vi "SendOracleRequest.vi"(8 "error in (no error)":errorcluster, 9 "Timeout":i32=5000, 10 "Report End Date":timestamp, 11 "Report Start Date":timestamp) -> (0 "error out":errorcluster, 3 "String":string)   [LabVIEW 2018, in "Controller.lvlib"]
uses:
  Controller.lvlib
  SRDataManagement_1.0/MainFrame/MainFrameLib.lvlib
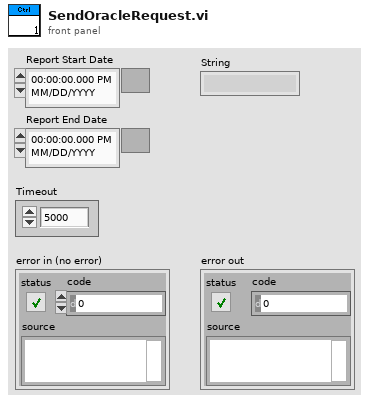
[diagram p1: front panel]
types:
  T1 = enum16{"Read", "Write", "ReadWrite", "BufferedRead", "BufferedReadWrite"}
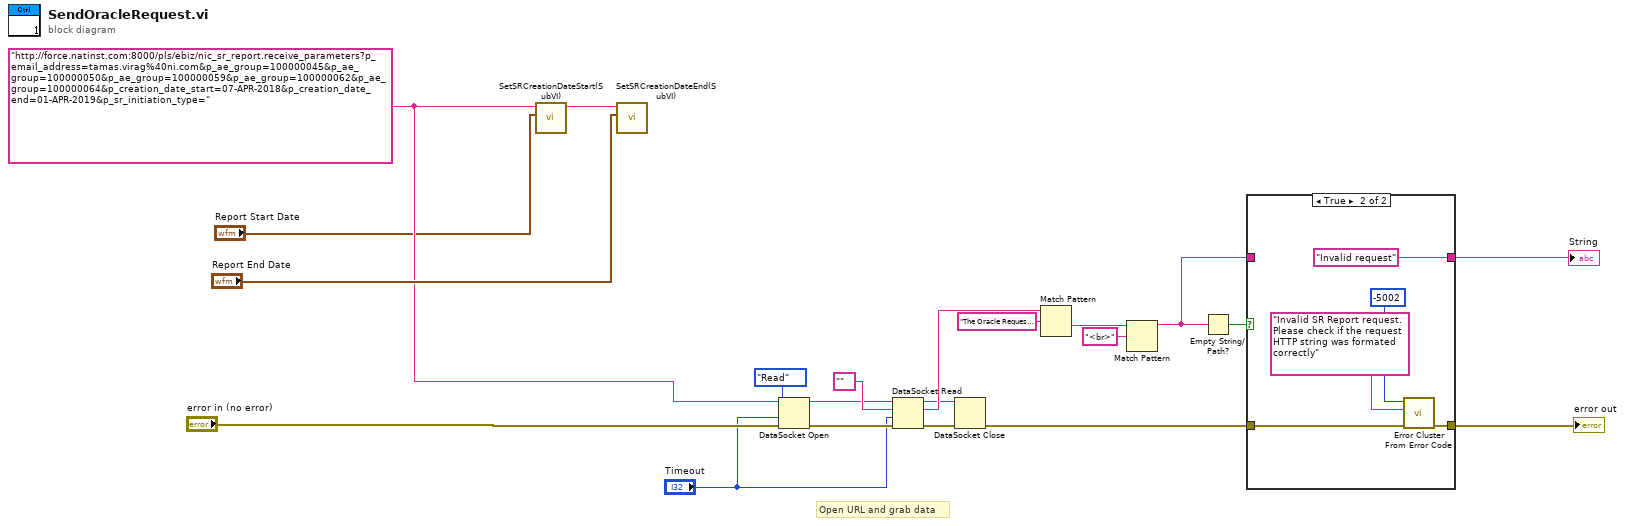
[diagram p0: block diagram]
diagram:
  w2 = "http://force.natinst.com:8000/pls/ebiz/nic_sr_report.receive_parameters?p_email_address=tamas.virag%40ni.com&p_ae_group=100000045&p_ae_group=100000050&p_ae_group=100000059&p_ae_group=100000062&p_ae_group=100000064&p_creation_date_start=07-APR-2018&p_creation_date_end=01-APR-2019&p_sr_initiation_type=" ("HTTP string")
  # "Open URL and grab data"
  n1 = call "SetSRCreationDateStart(SubVI).vi"("Date"="Report Start Date", "HTTP string"=w2) -> ("result string"=w16:string)  [unwired: 9 in]
  n2 = call "SetSRCreationDateEnd(SubVI).vi"("seconds since 1Jan1904"="Report End Date", "HTTP string in"=w16) -> ()  [unwired: 9 in, 1 out]
  n3 = DataSocket Open(8:"error in (no error)", 9:"Timeout", 10:T1."Read" ("mode"), 11:w2) -> (0:w8:errorcluster, 3:w7:refnum<k13>)
  n4 = DataSocket Read(8:w8, 9:"Timeout", 10:"", 11:w7) -> (0:w6:errorcluster, 2:w14:string, 3:w5:refnum<k13>)  [unwired: 1 in, 4 out]
  n5 = DataSocket Close(8:w6, 11:w5) -> (0:w19:errorcluster)  [unwired: 1 in, 1 out]
  n6 = Match Pattern(string=w14, regular expression="The Oracle Request ID for your report is ") -> (after substring=w12:string)  [unwired: 1 in, 3 out]
  n7 = Match Pattern(string=w12, regular expression="<br>") -> (before substring=w17:string)  [unwired: 1 in, 3 out]
  n8 = Empty String/Path?(string/path=w17) -> (empty?=w15:bool)
  n9 = case shown="True" w15 {
    tunnel: w17 -> [w23 _]
    tunnel: [w23 "Invalid request"] -> w18
    tunnel: w19 -> [w22 w27]
    tunnel: [w22 w25] -> w20
    frame False {
    }
    frame True {
      n10 = call <vilib>:"Error Cluster From Error Code.vi"("error in (no error)"=w27, "error message (\"\")"="Invalid SR Report request. Please check if the request HTTP string was formated correctly" ("error message (\"\")"), "error code (0)"=-5002) -> ("error out"=w25:errorcluster)  [unwired: 6 in]
    }
  }
  "error out" <- w20
  "String" <- w18
